vi "Create Type Data Clusters.vi"   [LabVIEW 2019, in "gRPC Template Creation Utility.lvlib"]
uses:
  gRPC Template Creation Utility.lvlib
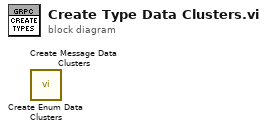
[diagram p0: block diagram]
diagram:
  n1 = call "Create Enum Data Clusters.vi"() -> ()  [unwired: 10 in, 2 out]
  n2 = call "Create Message Data Clusters.vi"() -> ()  [unwired: 10 in, 2 out]
